vi "Park (FXP).vi"(2 "Theta":fxp<+/-,32,1>, 3 "beta":fxp<+/-,32,4>, 4 "alpha":fxp<+/-,32,4>) -> (0 "q":fxp<+/-,32,4> format="%.30g", 1 "d":fxp<+/-,32,4> format="%.30g")   [LabVIEW 2025]
uses:
  <vilib>/rvi/FXPMathLib/FxpSinAndCos/subVIs/nifxpmath_SinAndCos_SimConfig.ctl
  <vilib>/rvi/FXPMathLib/FxpSinAndCos/simVIs/DllFxpSinAndCosTemp_sub.vi
  <vilib>/rvi/FXPMathLib/FxpSinAndCos/XNode/nifxpmath_SinAndCos.xnode
  <vilib>/rvi/FXPMathLib/FxpAdd/XNode/nifxpmath_Add.xnode
  <vilib>/rvi/FXPMathLib/sim/FxpSim.dll
  <vilib>/rvi/FXPMathLib/FxpMul/XNode/nifxpmath_Multiplier.xnode
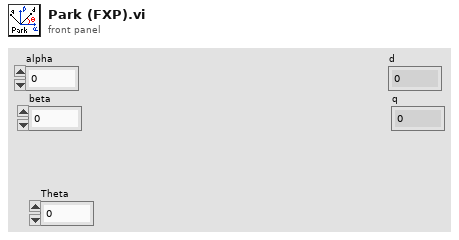
[diagram p1: front panel]
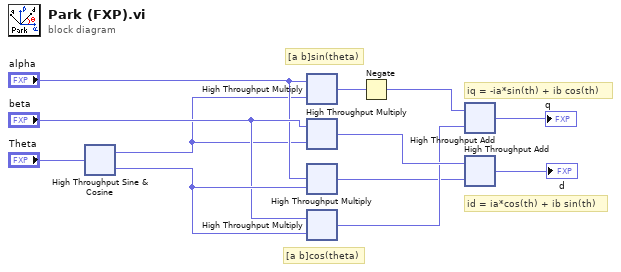
[diagram p0: block diagram]
diagram:
  # "id = ia*cos(th) + ib sin(th)"
  # "iq = -ia*sin(th) + ib cos(th)"
  # "[a b]cos(theta)"
  # "[a b]sin(theta)"
  n1 = xnode "High Throughput Sine & Cosine"("x (pi)"="Theta") -> ("sin(x)"=w3:fxp<+/-,16,2>, "cos(x)"=w12:fxp<+/-,16,2>)
  n2 = xnode "High Throughput Multiply"("x"="alpha", "y"=w3) -> ("x*y"=w4:fxp<+/-,32,4>)
  n3 = xnode "High Throughput Multiply"("x"="beta", "y"=w3) -> ("x*y"=w11:fxp<+/-,32,4>)
  n4 = xnode "High Throughput Multiply"("x"="alpha", "y"=w12) -> ("x*y"=w6:fxp<+/-,32,4>)
  n5 = xnode "High Throughput Multiply"("x"="beta", "y"=w12) -> ("x*y"=w8:fxp<+/-,32,4>)
  n6 = Negate(x=w4) -> (-x=w1:fxp<+/-,33,5>)
  n7 = xnode "High Throughput Add"("x"=w1, "y"=w8) -> ("x+y"=→"q":fxp<+/-,32,4>)
  n8 = xnode "High Throughput Add"("x"=w11, "y"=w6) -> ("x+y"=→"d":fxp<+/-,32,4>)
